vi "open ASI stage.vi"(8 "error in (no error)":errorcluster, 9 "timeout":u32=100, 10 "Baud rate":u32=115200, 11 "ASI stage":T1) -> (0 "error out":errorcluster, 3 "ASI stage out":T1)   [LabVIEW 2010]
uses:
  stage properties.ctl
  <vilib>/Instr/_visa.llb/VISA Flush IO Buffer Mask.ctl
  <vilib>/Instr/_visa.llb/VISA Configure Serial Port (Instr).vi
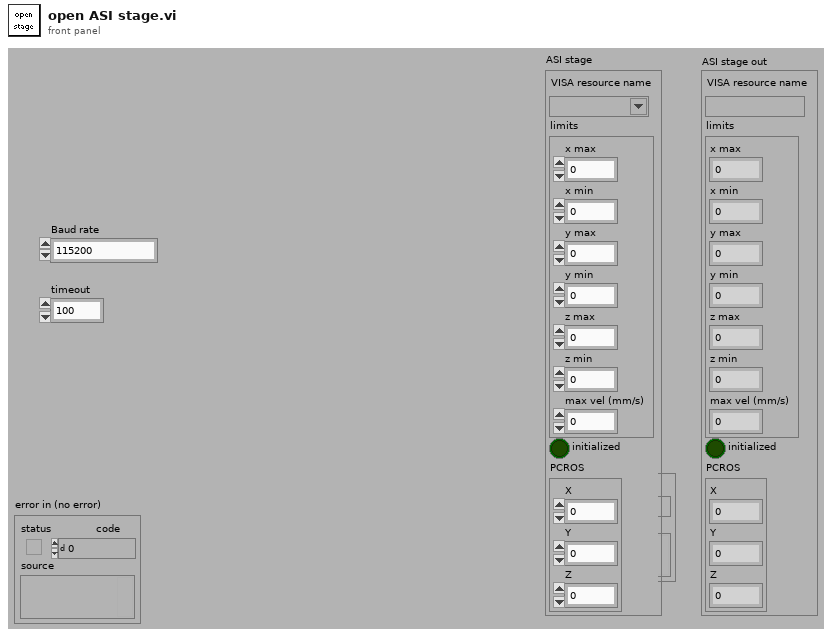
[diagram p1: front panel]
types:
  T1 = typedef "stage properties.ctl" = cluster{"VISA resource name":refnum<visa-resource-name>, "limits":cluster{"x max":dbl, "x min":dbl, "y max":dbl, "y min":dbl, "z max":dbl, "z min":dbl, "max vel (mm/s)":dbl}, "initialized":bool, "PCROS":cluster{"X":dbl, "Y":dbl, "Z":dbl}}
  T2 = typedef "VISA Flush IO Buffer Mask.ctl" = u16
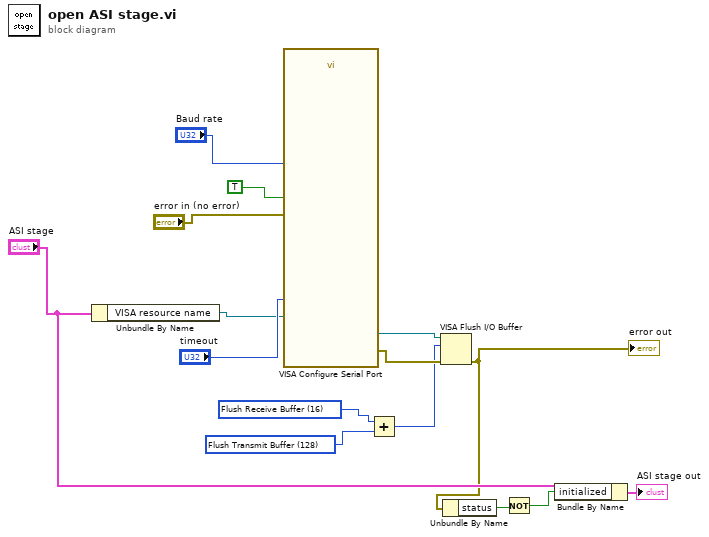
[diagram p0: block diagram]
diagram:
  w8 = T2 128 items=["Flush Receive Buffer"=16, "Write Transmit Buffer to Device"=32, "Flush Receive Buffer (No I/O)"=64, "Flush Transmit Buffer"=128] ("Mask")
  w7 = T2 16 items=["Flush Receive Buffer"=16, "Write Transmit Buffer to Device"=32, "Flush Receive Buffer (No I/O)"=64, "Flush Transmit Buffer"=128] ("Mask")
  n1 = Unbundle By Name("ASI stage") -> ("VISA resource name"=w11:refnum<visa-resource-name>)
  n2 = call-poly "VISA Configure Serial Port"("VISA resource name"=w11, "timeout (10sec)"="timeout", "Enable Termination\nChar (T)"=TRUE ("Enable Termination\nChar (T)"), "baud rate (9600)"="Baud rate", "error in (no error)"="error in (no error)") -> ("VISA resource name out"=w9:refnum<visa-resource-name>, "error out"=w10:errorcluster)  [unwired: 3 in, 6 out]
  n3 = Add(x=w7, y=w8) -> (x+y=w6:T2)
  n4 = VISA Flush I/O Buffer(VISA resource name=w9, mask (16)=w6, error in (no error)=w10) -> (error out=w4:errorcluster)  [unwired: 1 out]
  "error out" <- w4
  n5 = Unbundle By Name(w4) -> ("status"=w3:bool)
  n6 = Not(x=w3) -> (.not. x?=w2:bool)
  n7 = Bundle By Name(cluster="ASI stage", "initialized"=w2) -> (→"ASI stage out":T1)
